vi "FGV.vi"(1 "GetSetEnum":T2=enum."Get", 2 "ASIODataIn":T1={"Buffer Config"={"# buffers"=4, "Buffer size"=2048, "unit (ms)"=enum."Samples"}, "Format (44kHz, 16Bit, stereo)"={"Rate"=44100, "Bits"=16, "Channels"=2}, "Play"=FALSE, "Exit"=FALSE}) -> (0 "ASIODataOut":T1={"Buffer Config"={"# buffers"=4, "Buffer size"=2048, "unit (ms)"=enum."Samples"}, "Format (44kHz, 16Bit, stereo)"={"Rate"=44100, "Bits"=16, "Channels"=2}, "Play"=FALSE, "Exit"=FALSE})   [LabVIEW 2016]
uses:
  FGV/GetSetEnum.ctl
  FGV/ASIOData.ctl
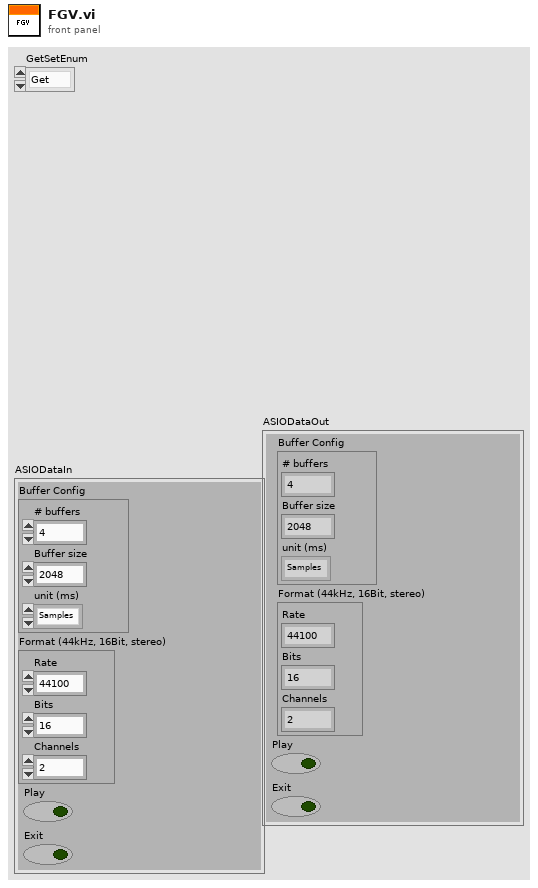
[diagram p1: front panel]
types:
  T1 = typedef "ASIOData.ctl" = cluster{"Buffer Config":cluster{"# buffers":i32, "Buffer size":i32, "unit (ms)":enum16{"time (ms)", "Samples"}}, "Format (44kHz, 16Bit, stereo)":cluster{"Rate":i32, "Bits":i32, "Channels":u32}, "Play":bool, "Exit":bool}
  T2 = typedef "GetSetEnum.ctl" = enum16{"Init", "Get", "Set"}
  T3 = cluster{"# buffers":i32, "Buffer size":i32, "unit (ms)":enum16{"time (ms)", "Samples"}}
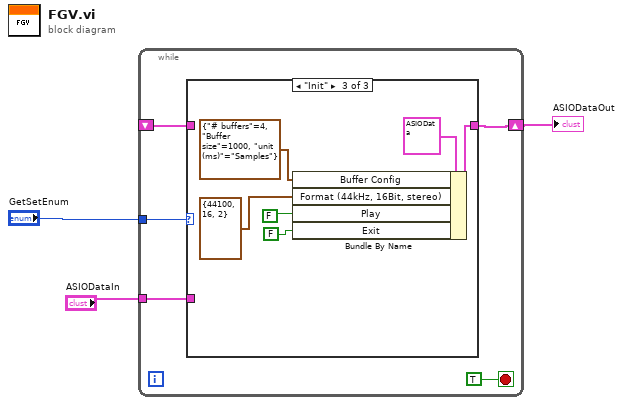
[diagram p0: block diagram]
diagram:
  n1 = while {
    tunnel: "GetSetEnum" -> [w7]
    shift-right: [w5] -> w1
    shift-left: _ -> [w6]
    tunnel: "ASIODataIn" -> [w4]
    stop <- TRUE stop-if-true
    n2 = case shown="\"Init\"" w7 {
      tunnel: w6 -> [w9 _ _]
      tunnel: [w9 w10 w15] -> w5
      tunnel: w4 -> [_ w10 _]
      frame "Get", Default {
      }
      frame "Set" {
      }
      frame "Init" {
        n3 = Bundle By Name(cluster=T1 {"Buffer Config"={"# buffers"=4, "Buffer size"=2048, "unit (ms)"=enum."Samples"}, "Format (44kHz, 16Bit, stereo)"={"Rate"=44100, "Bits"=16, "Channels"=2}, "Play"=FALSE, "Exit"=FALSE} ("ASIODataIn"), "Buffer Config"=T3 {"# buffers"=4, "Buffer size"=1000, "unit (ms)"=enum."Samples"}, "Format (44kHz, 16Bit, stereo)"=cluster{"Rate":i32, "Bits":i32, "Channels":u32} {"Rate"=44100, "Bits"=16, "Channels"=2}, "Play"=FALSE, "Exit"=FALSE) -> (w15:T1)
      }
    }
  }
  "ASIODataOut" <- w1
